vi "GetCCMTableData.vi"(11 "[[CMM Table 106]]":string[][](array[string])) -> ()   [LabVIEW 2018, in "Controller (Host).lvlib"]
uses:
  Controller (Host).lvlib
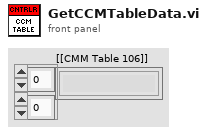
[diagram p1: front panel]
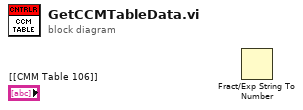
[diagram p0: block diagram]
diagram:
  n1 = Fract/Exp String To Number() -> ()  [unwired: 4 in, 2 out]
